vi "Calculate Mask Test Horizontal Offset Query.vi"(8 "error in":errorcluster, 11 "Instrument Handle In":i32) -> (0 "error out":errorcluster, 2 "Offset":dbl, 3 "Instrument Handle Out":i32)   [LabVIEW 8.6, in "ZTScopeM.lvlib"]
doc: "Returns the horizontal offset for generated masks"
uses:
  ZTScopeM.lvlib
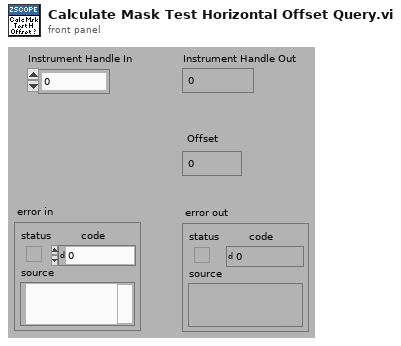
[diagram p1: front panel]
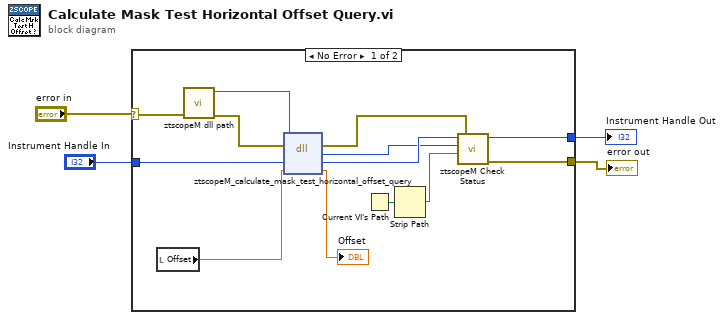
[diagram p0: block diagram]
diagram:
  n1 = case shown="No Error" "error in" {
    selector: "error in" -> [w8 w19]
    tunnel: [w12 w19] -> w1
    tunnel: "Instrument Handle In" -> [w17 w18]
    tunnel: [w11 w18] -> w3
    frame #0 {
      n2 = local read "Offset"() -> (w9:dbl)
      n3 = call "ztscopeM dll path.vi"("error in (no error)"=w8) -> ("error out"=w6:errorcluster, "<instrument>.dll path"=w7:path)  [unwired: 9 in]
      n4 = dll-call lib="C:/Program Files (x86)/National Instruments/LabVIEW 2013/instr.lib/ztscopem/ztscopeM.dll" fn="ztscopeM_calculate_mask_test_horizontal_offset_query"(path in=w7, error in=w6, "instrumentHandle"=w17, "offset"=w9) -> (error out=w5:errorcluster, w13:i32, "instrumentHandle"=w14:i32, "offset"=→"Offset":dbl)  [unwired: 1 in, 1 out]
      n5 = Current VI's Path() -> (path=w16:path)
      n6 = Strip Path(path=w16) -> (name=w15:string)  [unwired: 1 out]
      n7 = call "ztscopeM Check Status.vi"("error in"=w5, "name of VI"=w15, "status (return code)"=w13, "instrument handle in"=w14) -> ("error out"=w12:errorcluster, "instrument handle out"=w11:i32)  [unwired: 2 in]
    }
    frame #1 {
    }
  }
  "Instrument Handle Out" <- w3
  "error out" <- w1
